vi "Task Init.vi"(8 "error in (no error)":errorcluster, 11 "EventHandlerTask in":refnum<class "EventHandlerTask.lvclass">) -> (0 "error out":errorcluster, 3 "EventHandlerTask out":refnum<class "EventHandlerTask.lvclass">)   [LabVIEW 2020, in "Volatus.lvlib" / "EventHandlerTask.lvclass"]
uses:
  EventHandlerTask.lvclass
  EventHandlerTask.lvclass/EventHandlerTask.ctl
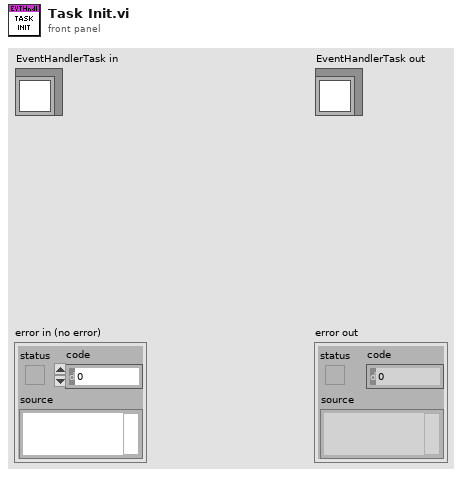
[diagram p1: front panel]
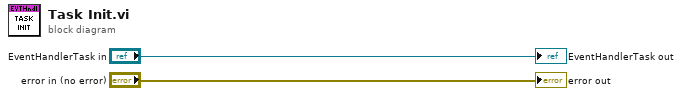
[diagram p0: block diagram]
diagram:
  "error out" <- "error in (no error)"
  "EventHandlerTask out" <- "EventHandlerTask in"
